vi "Insert Chan Group.vi"(5 "Insert to Prev Place? (T)":bool=TRUE, 7 "Timing Engine":T1, 8 "error in (no error)":errorcluster, 9 "ChanGroupPos":i32, 10 "ChanGrp to Add":refnum<class "ChanGrp.lvclass">, 11 "ChassisCfg in":refnum<class "ChassisCfg.lvclass">) -> (0 "error out":errorcluster, 1 "ChanGroupPos":i32, 3 "ChassisCfg out":refnum<class "ChassisCfg.lvclass">)   [LabVIEW 2012, in "Configuration Grandmaster.lvlib" / "ChassisCfg.lvclass"]
uses:
  ChassisCfg.lvclass
  Class Chan Group/ChanGrp.lvclass
  Common/Controls/TE_Designator.ctl
  ChassisCfg.lvclass/ChassisCfg.ctl
  Class Timing Group/TimingGrp.lvclass
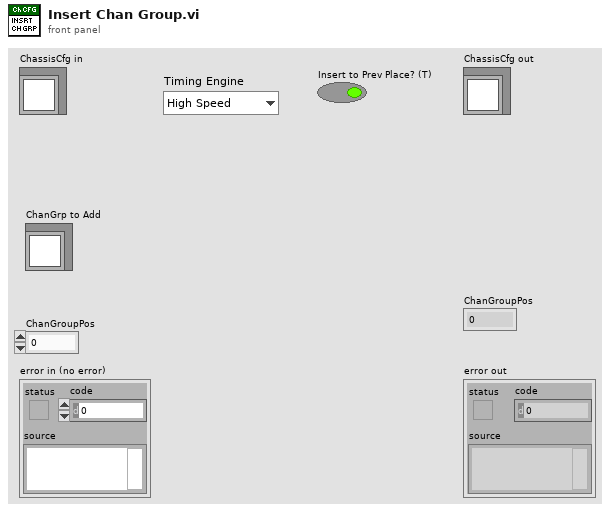
[diagram p1: front panel]
types:
  T1 = typedef "TE_Designator.ctl" = enum16{"High Speed", "Low Speed"}
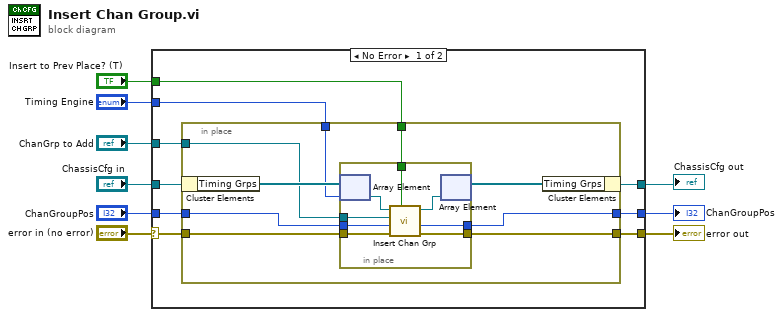
[diagram p0: block diagram]
diagram:
  n1 = case shown="No Error" "error in (no error)" {
    selector: "error in (no error)" -> [w12 w36]
    tunnel: [w18 w36] -> w9
    tunnel: "ChassisCfg in" -> [w17 w38]
    tunnel: [w16 w38] -> w7
    tunnel: "ChanGrp to Add" -> [w15 _]
    tunnel: "ChanGroupPos" -> [w14 w37]
    tunnel: [w13 w37] -> w4
    tunnel: "Insert to Prev Place? (T)" -> [w11 _]
    tunnel: "Timing Engine" -> [w10 _]
    frame No Error {
      n2 = in-place {
        in-place-border: w12 -> [w27]
        in-place-border: [w26] -> w18
        in-place-border: w15 -> [w23]
        in-place-border: w14 -> [w20]
        in-place-border: [w22] -> w13
        in-place-border: w11 -> [w21]
        in-place-border: w10 -> [w19]
        n3 = in-place-cluster #1(w17) -> ("Timing Grps"=w24:refnum<class "TimingGrp.lvclass">[])
        n4 = in-place {
          in-place-border: [w35] -> w22
          in-place-border: w23 -> [w34]
          in-place-border: w27 -> [w33]
          in-place-border: [w32] -> w26
          in-place-border: w20 -> [w31]
          in-place-border: w21 -> [w30]
          n5 = in-place-array #2(w24, w19) -> (w29:refnum<class "TimingGrp.lvclass">)
          n6 = call "Insert Chan Grp.vi"("Insert to Prev Place? (T)"=w30, "error in (no error)"=w33, "ChanGroupPos"=w31, "ChanGrp to Add"=w34, "TimingGrp in"=w29) -> ("error out"=w32:errorcluster, "ChanGroupPos"=w35:i32, "TimingGrp out"=w28:refnum<class "TimingGrp.lvclass">)  [unwired: 4 in]
          n7 = in-place-array #2(w28) -> (w25:refnum<class "TimingGrp.lvclass">[])  [unwired: 1 out]
        }
        n8 = in-place-cluster #1("Timing Grps"=w25) -> (w16:refnum<class "ChassisCfg.lvclass">)
      }
    }
    frame Error {
    }
  }
  "error out" <- w9
  "ChassisCfg out" <- w7
  "ChanGroupPos" <- w4
